vi "Emit.vi"(8 "error in (no error)":errorcluster, 10 "response":T1, 11 "QueueResponder in":refnum<class "QueueResponder.lvclass">) -> (0 "error out":errorcluster, 3 "QueueResponder out":refnum<class "QueueResponder.lvclass">)   [LabVIEW 2013, in "QueueResponder.lvclass"]
doc: "Emit a response to the owning application"
uses:
  QueueResponder.lvclass
  response.ctl
  driver_status.ctl
  QueueResponder.lvclass/QueueResponder.ctl
  BaseResponder/BaseResponder.lvclass
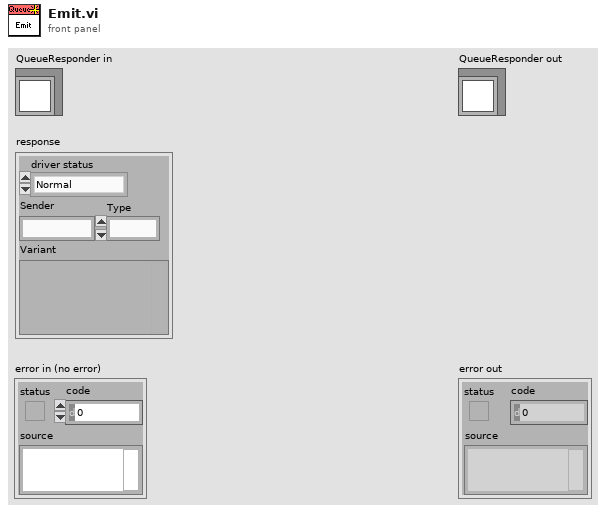
[diagram p1: front panel]
types:
  T1 = typedef "response.ctl" = cluster{"driver status":T2, "Sender":string, "Type":i32, "Variant":variant}
  T2 = typedef "driver_status.ctl" = enum16{"Normal", "Startup", "Connection lost", "Reconnected", "Timeout", "Idle", "Busy"}
  T3 = typedef "response queue.ctl" = refnum<queue>
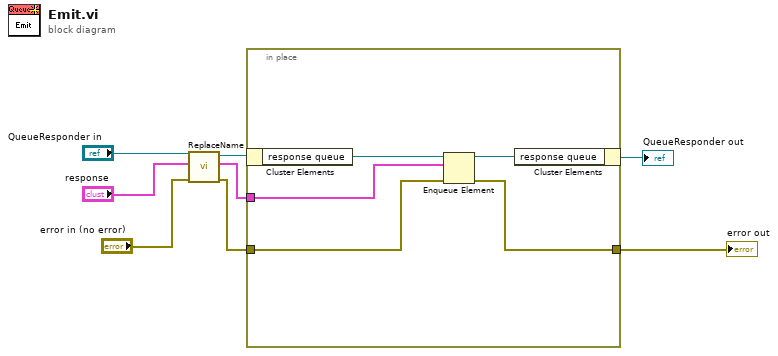
[diagram p0: block diagram]
diagram:
  n1 = call "ReplaceName.vi"("error in (no error)"="error in (no error)", "response"="response", "BaseResponder in"="QueueResponder in") -> ("error out"=w1:errorcluster, "response out"=w2:T1, "BaseResponder out"=w5:refnum<class "QueueResponder.lvclass">)  [unwired: 6 in]
  n2 = in-place "In Place Element Structure" {
    in-place-border: w2 -> [w11]
    in-place-border: w1 -> [w10]
    in-place-border: [w9] -> w7
    n3 = in-place-cluster #1(w5) -> ("response queue"=w13:T3)
    n4 = Enqueue Element(queue=w13, element=w11, error in (no error)=w10) -> (queue out=w12:T3, error out=w9:errorcluster)  [unwired: 1 in, 1 out]
    n5 = in-place-cluster #1("response queue"=w12) -> (→"QueueResponder out":refnum<class "QueueResponder.lvclass">)
  }
  "error out" <- w7
